vi "Write Data.vi"(3 "error in":errorcluster, 4 "NodeIds":T2[](array[typedef]), 5 "OPC UA server refnum":T1) -> (0 "error out":errorcluster)   [LabVIEW 2020]
uses:
  <vilib>/OPCUA/NI OPC UA Server.lvlib
  <vilib>/OPCUA/server/Write Double.vi
  <vilib>/OPCUA/controls/NodeId.ctl
  <vilib>/OPCUA/controls/OPC UA Server Refnum.ctl
panel:
  in  "Value":dbl
  in  "Node Id":u16(ring) items=["ns=2;s=Nodes.Temperature", "ns=2;s=Nodes.Pressure", "ns=2;s=Nodes.Flow"]
  in  "OK Button":bool
  in  "Cancel Button":bool
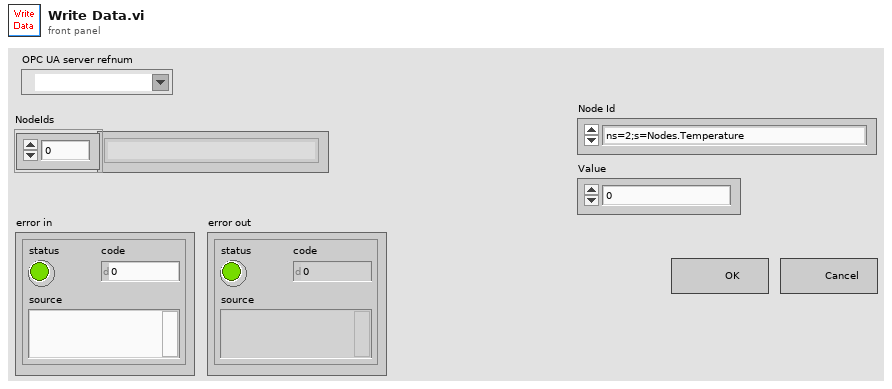
[diagram p1: front panel]
types:
  T1 = typedef "OPC UA Server Refnum.ctl" = refnum<k21>
  T2 = typedef "NodeId.ctl" = string
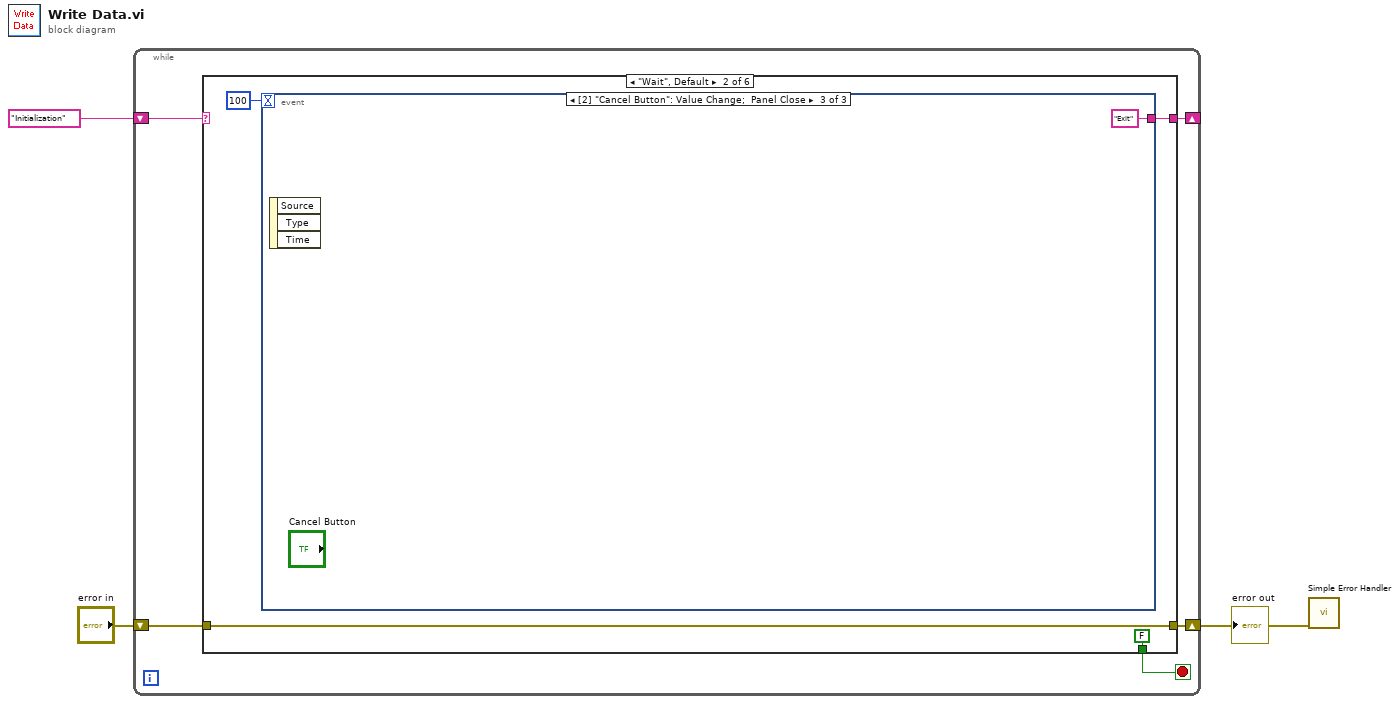
[diagram p0: block diagram]
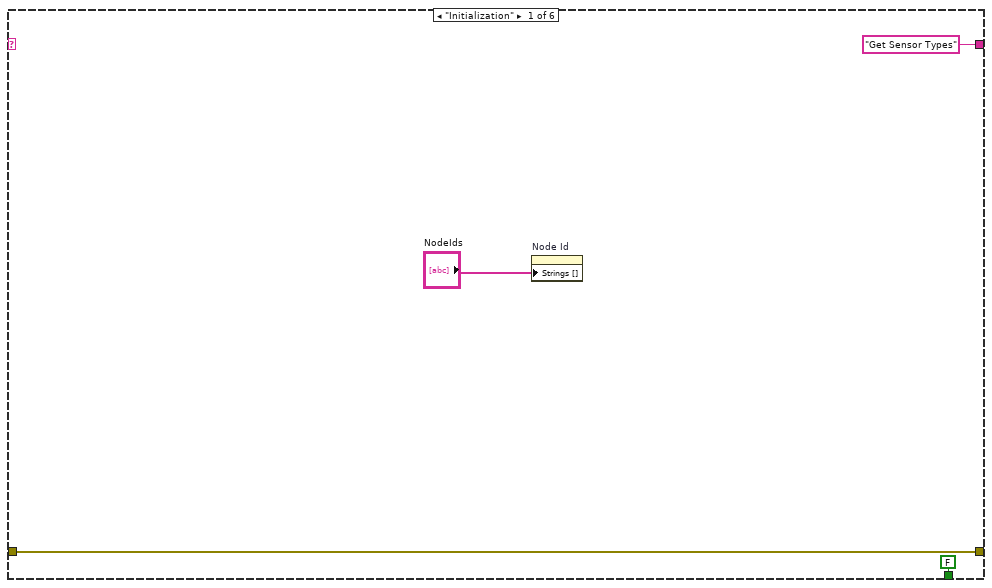
[diagram p2: hidden frame]
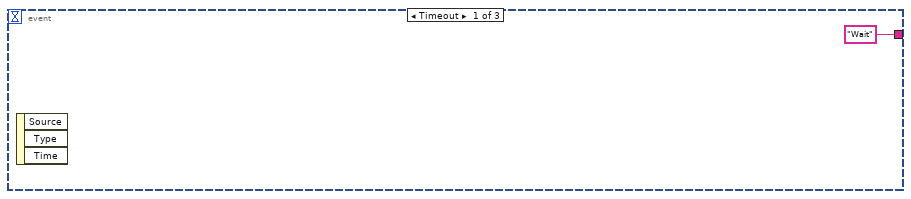
[diagram p3: hidden frame]
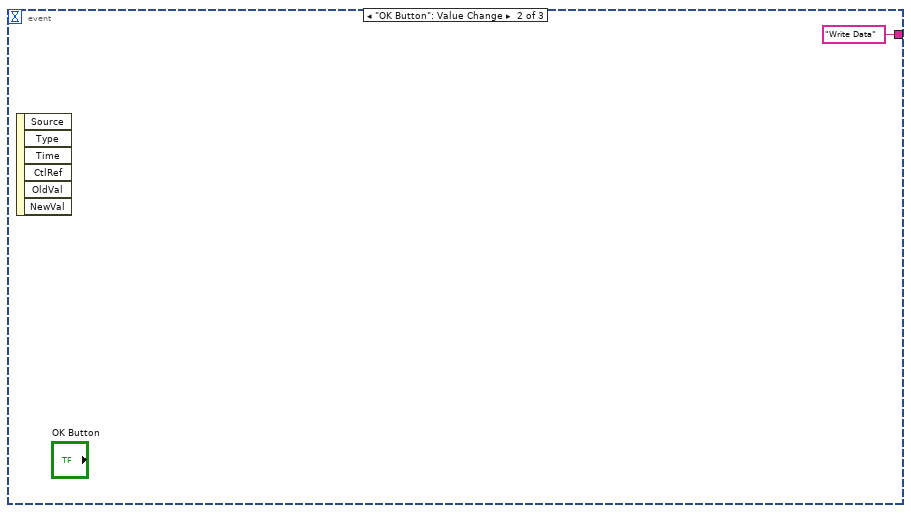
[diagram p4: hidden frame]
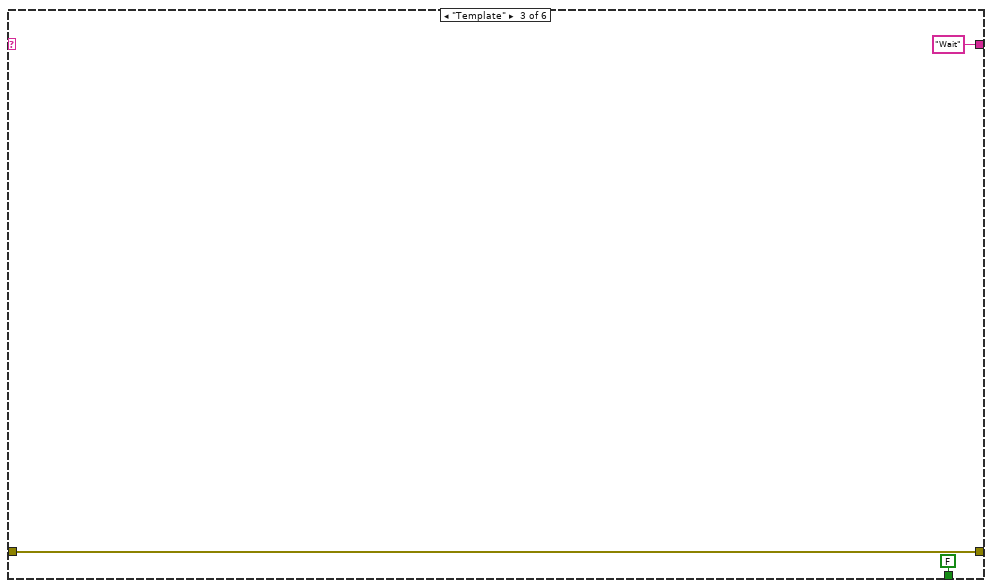
[diagram p5: hidden frame]
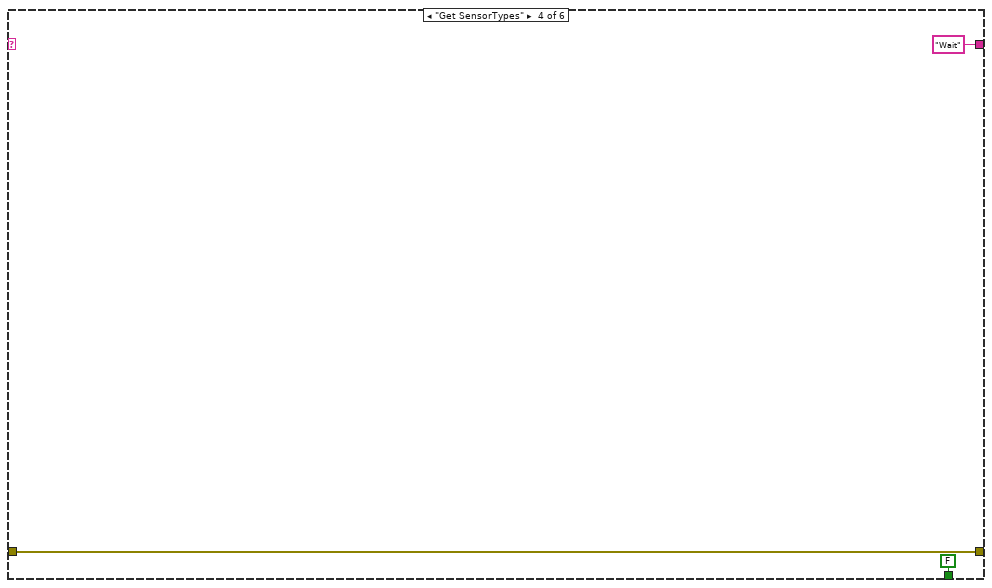
[diagram p6: hidden frame]
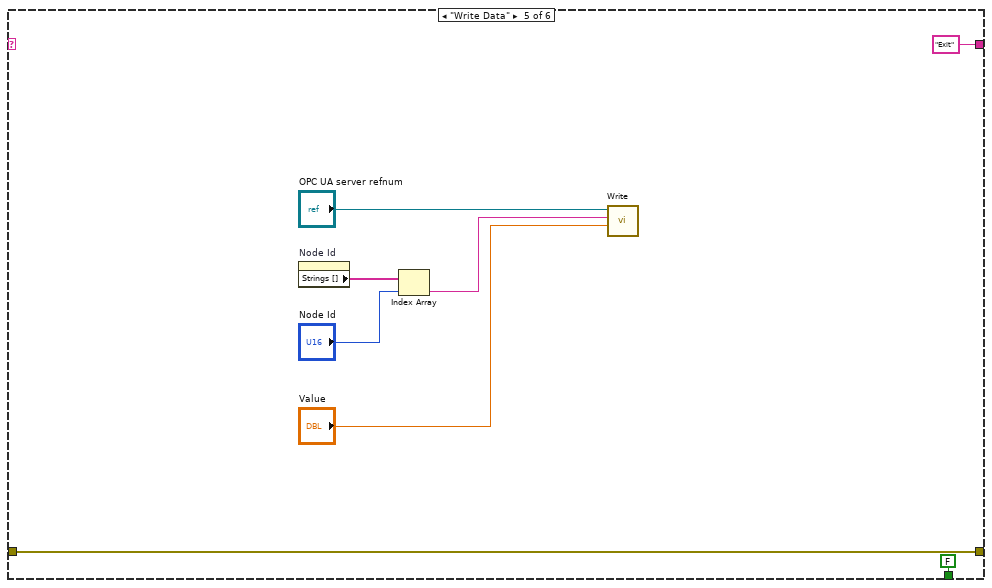
[diagram p7: hidden frame]
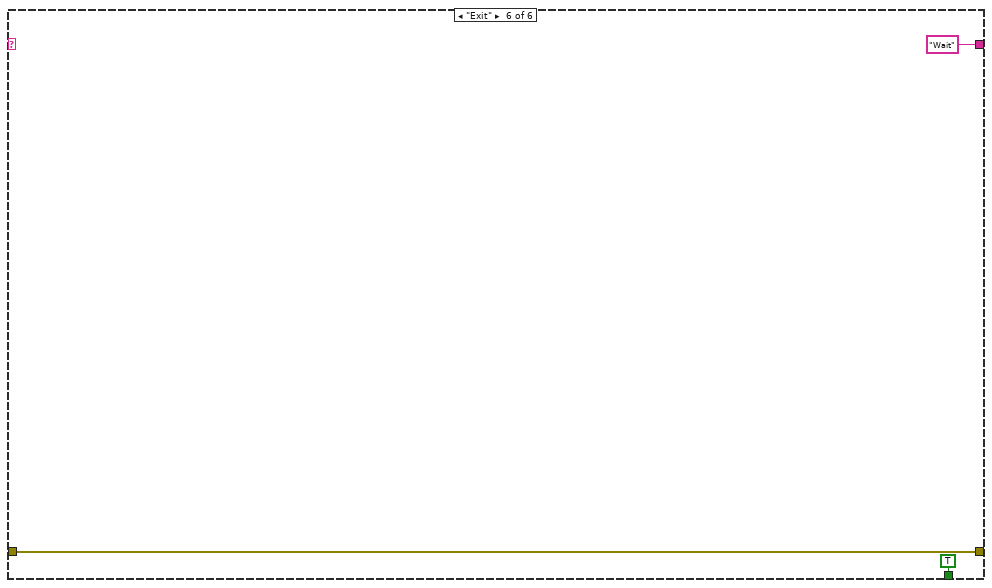
[diagram p8: hidden frame]
diagram:
  n1 = while {
    shift-right: [w7] -> _
    shift-left: "Initialization" -> [w8]
    shift-right: [w4] -> w1
    shift-left: "error in" -> [w5]
    stop <- w6 stop-if-true
    n2 = case shown="\"Wait\", Default" w8 {
      tunnel: ["Get Sensor Types" w14 "Wait" "Wait" "Exit" "Wait"] -> w7
      tunnel: [FALSE FALSE FALSE FALSE FALSE TRUE] -> w6
      tunnel: w5 -> [w10 w13 w20 w23 w31 w34]
      tunnel: [w10 w13 w20 w23 w31 w34] -> w4
      frame "Initialization" {
        n3 = property on="Node Id" class="Ring (strict)"("Strings []"="NodeIds") -> ()  [unwired: 2 in, 2 out]
      }
      frame "Wait", Default {
        n4 = event shown="[2] \"Cancel Button\": Value Change;  Panel Close" {
          selector: _ -> [_ _ _]
          dyn-events: _ -> [_ _ _]
          timeout: 100 ("ms") -> [_ _ _]
          tunnel: ["Wait" "Write Data" "Exit"] -> w14
          event Timeout {
            n5 = event-data() -> ()  [unwired: 1 in, 3 out]
          }
          event "OK Button": Value Change {
            n6 = event-data() -> ()  [unwired: 1 in, 6 out]
          }
          event "Cancel Button": Value Change; Panel Close {
            n7 = event-data() -> ()  [unwired: 1 in, 3 out]
          }
        }
      }
      frame "Template" {
      }
      frame "Get SensorTypes" {
      }
      frame "Write Data" {
        n8 = property on="Node Id" class="Ring (strict)"() -> ("Strings []"=w28:string[])  [unwired: 2 in, 2 out]
        n9 = Index Array "Index Array"(array=w28, index="Node Id") -> (element=w26:string)
        n10 = call-poly <vilib>:"Write.vi"("value"="Value", "node ID"=w26, "OPC UA server refnum in"="OPC UA server refnum") -> ()  [unwired: 6 in, 3 out]
      }
      frame "Exit" {
      }
    }
  }
  "error out" <- w1
  n11 = call <vilib>:"Simple Error Handler.vi"("error in (no error)"=w1) -> ()  [unwired: 4 in, 5 out]
